vi "Read Edgesense params.vi"(8 "error in (no error)":errorcluster, 11 "AlessiRel6100 in":refnum<class "AlessiRel6100.lvclass">) -> (0 "error out":errorcluster, 2 "Edgesense params":T1={"touchdown height [µm]"=0, "search band [µm]"=100, "speed [µm/step]"=10, "overdrive [µm]"=30}, 3 "AlessiRel6100 out":refnum<class "AlessiRel6100.lvclass">)   [LabVIEW 2013, in "AlessiRel6100.lvclass"]
uses:
  AlessiRel6100.lvclass
  AlessiRel6100.lvclass/AlessiRel6100.ctl
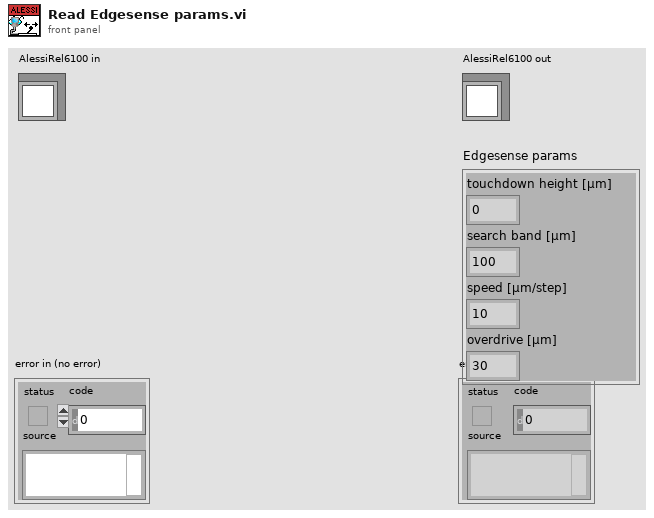
[diagram p1: front panel]
types:
  T1 = cluster{"touchdown height [µm]":i32, "search band [µm]":u32, "speed [µm/step]":u32, "overdrive [µm]":u32}
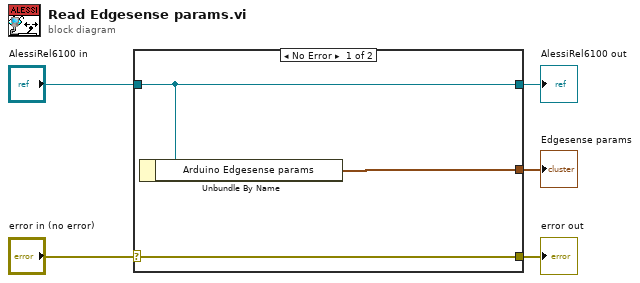
[diagram p0: block diagram]
diagram:
  n1 = case shown="No Error" "error in (no error)" {
    selector: "error in (no error)" -> [w8 w9]
    tunnel: [w8 w9] -> w4
    tunnel: [w7 w10] -> w2
    tunnel: "AlessiRel6100 in" -> [w7 w10]
    tunnel: [w6 _] -> w1
    frame No Error {
      n2 = Unbundle By Name(w7) -> ("Arduino Edgesense params"=w6:T1)
    }
    frame Error {
    }
  }
  "error out" <- w4
  "AlessiRel6100 out" <- w2
  "Edgesense params" <- w1
